vi "Perform Action.vi"(8 "error in":errorcluster, 10 "Input":variant, 11 "AI Voltage DAQmx Cont CFG Simulated in":refnum<class "AI Voltage DAQmx Cont CFG Simulated.lvclass">) -> (0 "error out":errorcluster, 2 "Output":variant, 3 "AI Voltage DAQmx Cont CFG Simulated out":refnum<class "AI Voltage DAQmx Cont CFG Simulated.lvclass">)   [LabVIEW 2024, in "DAQmx Simulated CFGs.lvlib" / "AI Voltage DAQmx Cont CFG Simulated.lvclass"]
uses:
  AI Voltage DAQmx Cont CFG Simulated.lvclass
  DAQmx BufferLastReadsDBL/DAQmx BufferLastReadsDBL.lvclass/DAQmx BufferLastReadsDBL.ctl
  0cc4d47a-a0da-4a28-b8ba-3adaf38567aa.vi
  <vilib>/JDP Science/JSONtext/Find Item.vi
  <vilib>/JDP Science/JSONtext/Next JSON Value.vi
  <vilib>/JDP Science/JSONtext/String Subset.vi
  <vilib>/JDP Science/JSONtext/Parsing/Advance past next JSON Value (inlined COPY).vi
  <vilib>/JDP Science/JSONtext/Parsing/Advance past whitespace.vi
  <vilib>/JDP Science/JSONtext/Parsing/Advance past String.vi
  <vilib>/JDP Science/JSONtext/Parsing/Advance past Number.vi
  <vilib>/JDP Science/JSONtext/Parsing/Advance past Line Ending.vi
  <vilib>/JDP Science/JSONtext/Parsing/Parse Full Path or Item Name.vi
  <vilib>/JDP Science/JSONtext/Parsing/Advance past Array.vi
  <vilib>/JDP Science/JSONtext/Parsing/Advance past Object.vi
  <vilib>/JDP Science/JSONtext/support/Error Cluster From Code.vi
  <vilib>/JDP Science/JSONtext/Offset/Find Item Locations by Path.vi
  <vilib>/JDP Science/JSONtext/JSON text to Variant.vi
  <vilib>/JDP Science/JSONtext/LVClass Serializer/JSONtext LVClass Serializer.lvclass
  DAQmx BufferLastReadsDBL/DAQmx BufferLastReadsDBL.lvclass
  Buffers/BufferLastReadingsDBL/BufferLastReadsDBL.lvclass
  Configurations/CFG JSON/CFG JSON.lvclass
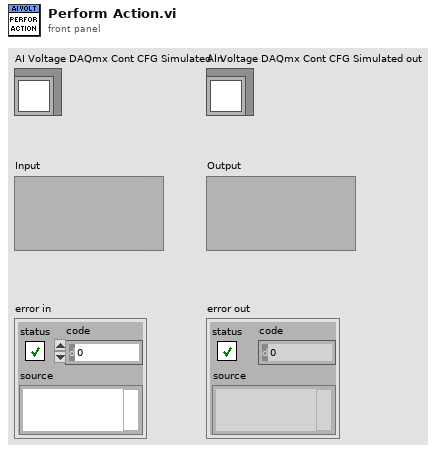
[diagram p1: front panel]
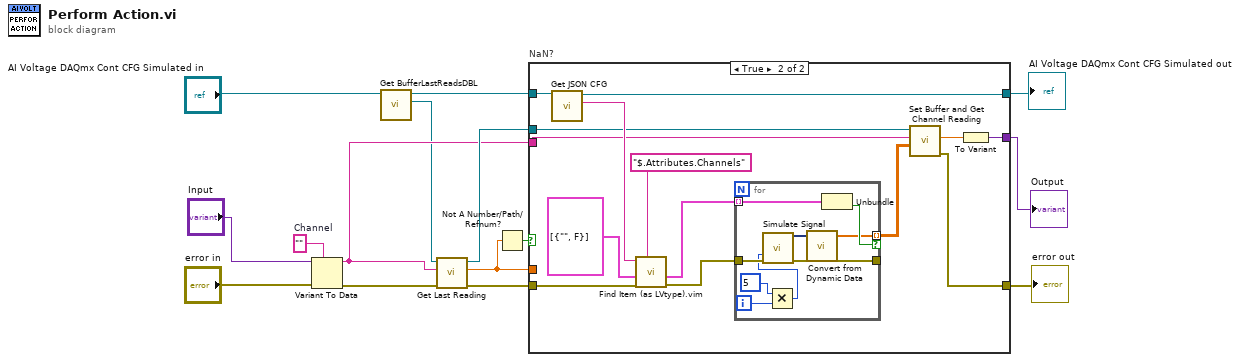
[diagram p0: block diagram]
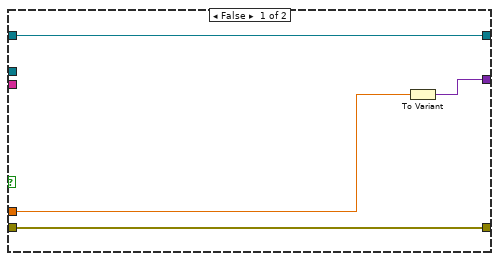
[diagram p2: hidden frame]
diagram:
  w11 = ""  # Channel
  n1 = Variant To Data(error in="error in", type=w11, Variant="Input") -> (data=w9:string, error out=w10:errorcluster)
  n2 = call "Get BufferLastReadsDBL.vi"("DAQmx BufferLastReadsDBL in"="AI Voltage DAQmx Cont CFG Simulated in") -> ("BufferLastReadsDBL.lvclass"=w7:refnum<class "BufferLastReadsDBL.lvclass">, "DAQmx BufferLastReadsDBL out"=w8:refnum<class "AI Voltage DAQmx Cont CFG Simulated.lvclass">)  [unwired: 9 in]
  n3 = call "Get Last Reading.vi"("error in"=w10, "Channel"=w9, "BufferLastReadingsDBL in"=w7) -> ("error out"=w13:errorcluster, "Reading"=w14:dbl, "BufferLastReadingsDBL out"=w12:refnum<class "BufferLastReadsDBL.lvclass">)  [unwired: 6 in]
  n4 = Not A Number/Path/Refnum?(number/path/refnum=w14) -> (NaN/Path/Refnum?=w15:bool)
  n5 = case "NaN?" shown="True" w15 {
    tunnel: [w16 w33] -> w1
    tunnel: [w17 w27] -> w3
    tunnel: w8 -> [w17 w28]
    tunnel: w12 -> [_ w26]
    tunnel: [w18 w32] -> w2
    tunnel: w14 -> [w19 _]
    tunnel: w13 -> [w16 w24]
    tunnel: w9 -> [_ w20]
    frame False {
      n6 = To Variant(anything=w19) -> (Variant=w18:variant)
    }
    frame True {
      n7 = call "Get JSON CFG.vi"("CFG JSON in"=w28) -> ("<JSON> CFG"=w30:string, "CFG JSON out"=w27:refnum<class "AI Voltage DAQmx Cont CFG Simulated.lvclass">)  [unwired: 9 in]
      n8 = call "Find Item (as LVtype).vim"("$Path or Item Name"="$.Attributes.Channels", "error in (no error)"=w24, "Data Type and Default Value"=cluster{"Name":string, "Enabled":bool}[] [{"Name"="", "Enabled"=FALSE}], "JSON"=w30) -> ("error out"=w23:errorcluster, "Data"=w22:cluster{"Name":string, "Enabled":bool}[])  [unwired: 4 in, 2 out]
      n9 = for {
        tunnel: w22 -> [w42] mode=indexing
        tunnel: w23 -> [w41]
        tunnel: [w40] -> _
        tunnel: [w35] -> w21 mode=indexing if=w39
        i -> [w38]
        n10 = Multiply(x=5, y=w38) -> (x*y=w34:i32)
        n11 = call "Simulate Signal"("Phase"=w34, "error in (no error)"=w41) -> ("Sine with Uniform Noise"=w36:dynamicdata, "error out"=w40:errorcluster)  [unwired: 12 in]
        n12 = call "Convert from Dynamic Data"("Dynamic Data Type"=w36) -> ("Array"=w35:dbl[])  [unwired: 3 in]
        n13 = Unbundle(w42) -> ("Enabled"=w39:bool)  [unwired: 1 out]
      }
      n14 = call "Set Buffer and Get Channel Reading.vi"("Readings"=w21, "Channel Ident"=w20, "BufferLastReadingsDBL in"=w26) -> ("error out"=w33:errorcluster, "Reading"=w31:dbl)  [unwired: 6 in, 1 out]
      n15 = To Variant(anything=w31) -> (Variant=w32:variant)
    }
  }
  "error out" <- w1
  "AI Voltage DAQmx Cont CFG Simulated out" <- w3
  "Output" <- w2
